vi "main.vi"() -> ()   [LabVIEW 2020]
uses:
  Generator.xctl
  Multimetr.xctl
panel:
  out "Coarse":dbl
  out "Fine":dbl
  in  "stop":bool
  out "Woltomierz":cluster{"Data":dbl, "Power":bool}(xcontrol)
  out "Amperomierz":cluster{"Data":dbl, "Power":bool}(xcontrol)
  in  "Generator":T3(xcontrol)
  out "P1":u16(ring)
  in  "C 2":bool
  in  "C1":bool
  out "P5":u16(ring)
  out "P4":u16(ring)
  out "P2":u16(ring)
  out "P3":u16(ring)
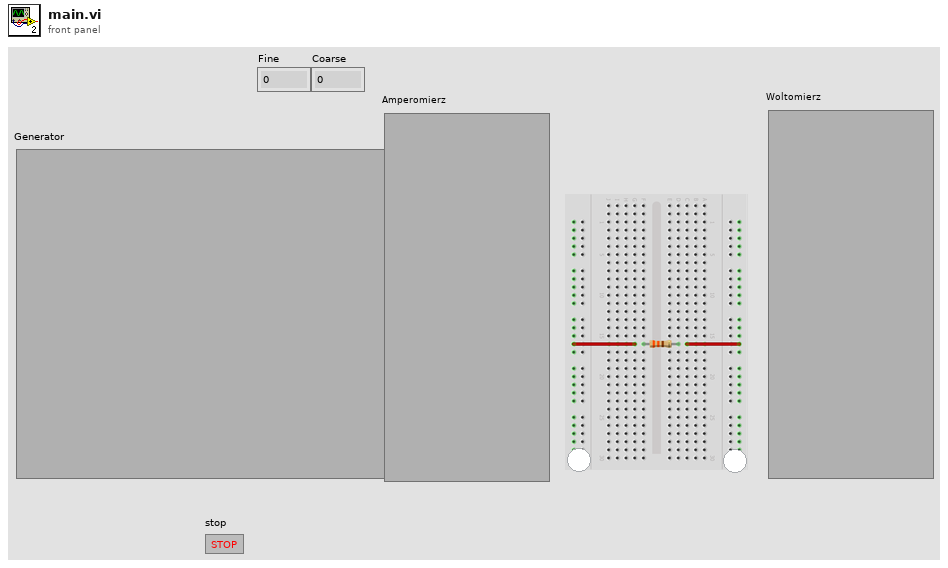
[diagram p1: front panel]
types:
  T1 = typedef "Power Ecran.ctl" = string
  T2 = typedef "Ecran data.ctl" = dbl
  T3 = cluster{"Data":dbl, "+":bool, "-":bool, "Output":bool, "Power ":bool, "Ecran Power":T1, "Ekran data":T2, "Coarse":dbl, "Fine":dbl}
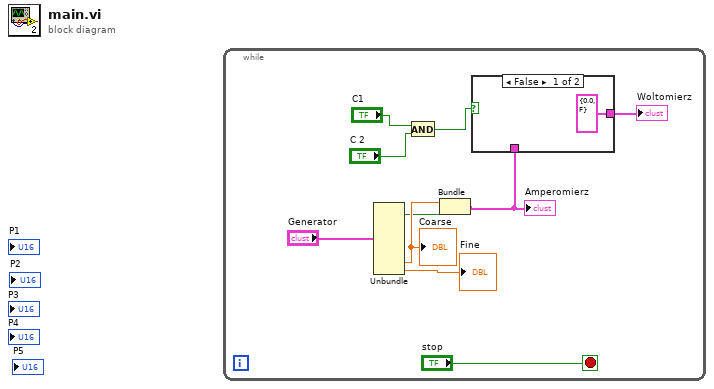
[diagram p0: block diagram]
diagram:
  n1 = while {
    stop <- "stop" stop-if-true
    n2 = Unbundle("Generator") -> ("+"=w7:bool, "Coarse"=w8:dbl, "Fine"=→"Fine":dbl)  [unwired: 6 out]
    "Coarse" <- w8
    n3 = And(x="C1", y="C 2") -> (x .and. y?=w3:bool)
    n4 = Bundle("Coarse"=w8, "+"=w7) -> (w1:cluster{"Coarse":dbl, "+":bool})  [unwired: 1 in]
    "Amperomierz" <- w1
    n5 = case shown="False" w3 {
      tunnel: [cluster{"Coarse":dbl, "+":bool} {"Coarse"=0.0, "+"=FALSE} w12] -> w2
      tunnel: w1 -> [_ w12]
      frame False {
      }
      frame True {
      }
    }
    "Woltomierz" <- w2
  }
